vi "产品高低配.vi"(4 "后":string=">", 5 "前":string="<", 6 "低配":string="低配", 7 "高配":string="高配", 9 "选择":i16) -> (0 "颜色":u32(colorbox), 1 "产品名称":string, 2 "物料编号":string, 3 "高低配":i16)   [LabVIEW 2018]
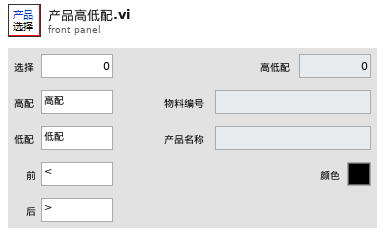
[diagram p1: front panel]
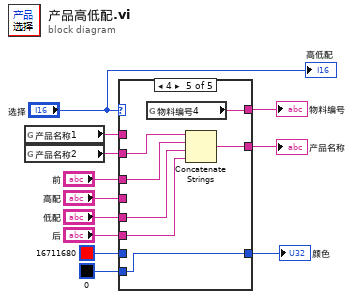
[diagram p0: block diagram]
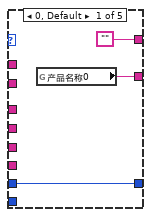
[diagram p2: hidden frame]
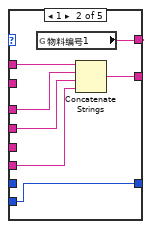
[diagram p3: hidden frame]
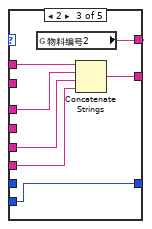
[diagram p4: hidden frame]
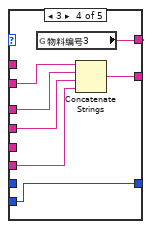
[diagram p5: hidden frame]
diagram:
  n1 = global read "全局 1.vi" "产品名称1"() -> (w12:string)
  n2 = global read "全局 1.vi" "产品名称2"() -> (w11:string)
  n3 = case shown="4" "选择" {
    tunnel: w12 -> [_ w21 w28 _ _]
    tunnel: w11 -> [_ _ _ w32 w39]
    tunnel: ["" w22 w29 w36 w43] -> w10
    tunnel: "高配" -> [_ w18 _ w31 _]
    tunnel: [w14 w20 w27 w35 w42] -> w8
    tunnel: "低配" -> [_ _ w24 _ w38]
    tunnel: "前" -> [_ w19 w26 w34 w41]
    tunnel: "后" -> [_ w17 w25 w33 w40]
    tunnel: u32 16711680 -> [w13 _ _ _ _]
    tunnel: u32 0 -> [_ w16 w23 w30 w37]
    tunnel: [w13 w16 w23 w30 w37] -> w1
    frame 0, Default {
      n4 = global read "全局 1.vi" "产品名称0"() -> (w14:string)
    }
    frame 1 {
      n5 = global read "全局 1.vi" "物料编号1"() -> (w22:string)
      n6 = Concatenate Strings(w21, w19, w18, w17) -> (w20:string)
    }
    frame 2 {
      n7 = global read "全局 1.vi" "物料编号2"() -> (w29:string)
      n8 = Concatenate Strings(w28, w26, w24, w25) -> (w27:string)
    }
    frame 3 {
      n9 = global read "全局 1.vi" "物料编号3"() -> (w36:string)
      n10 = Concatenate Strings(w32, w34, w31, w33) -> (w35:string)
    }
    frame 4 {
      n11 = global read "全局 1.vi" "物料编号4"() -> (w43:string)
      n12 = Concatenate Strings(w39, w41, w38, w40) -> (w42:string)
    }
  }
  "物料编号" <- w10
  "产品名称" <- w8
  "颜色" <- w1
  "高低配" <- "选择"
